vi "array -- find interval - real.vi"(8 "number":dbl, 11 "array":dbl[](array[numeric])=[10.0, 20.0, 56.0, 92.0, 120.0, 183.0, 194.0, 310.0]) -> (0 "omega plus (kHz)":dbl, 1 "omega zero (kHz)":dbl, 2 "omega minus (kHz)":dbl, 3 "out of range?":bool, 4 "closest element index":i32, 5 "exact match ?":bool)   [LabVIEW 2015]
uses:
  comparison control.ctl
  Q - not nan -- real.vi
panel:
  out "selector":T1
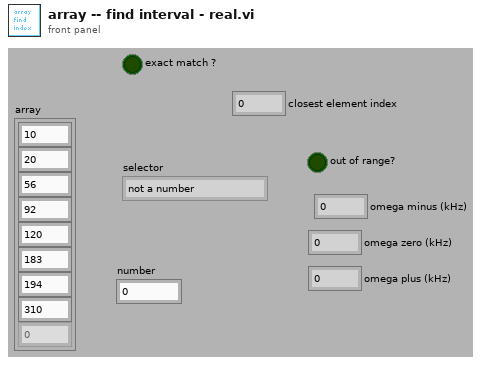
[diagram p1: front panel]
types:
  T1 = typedef "comparison control.ctl" = enum16{"not a number", "above", "in range", "below"}
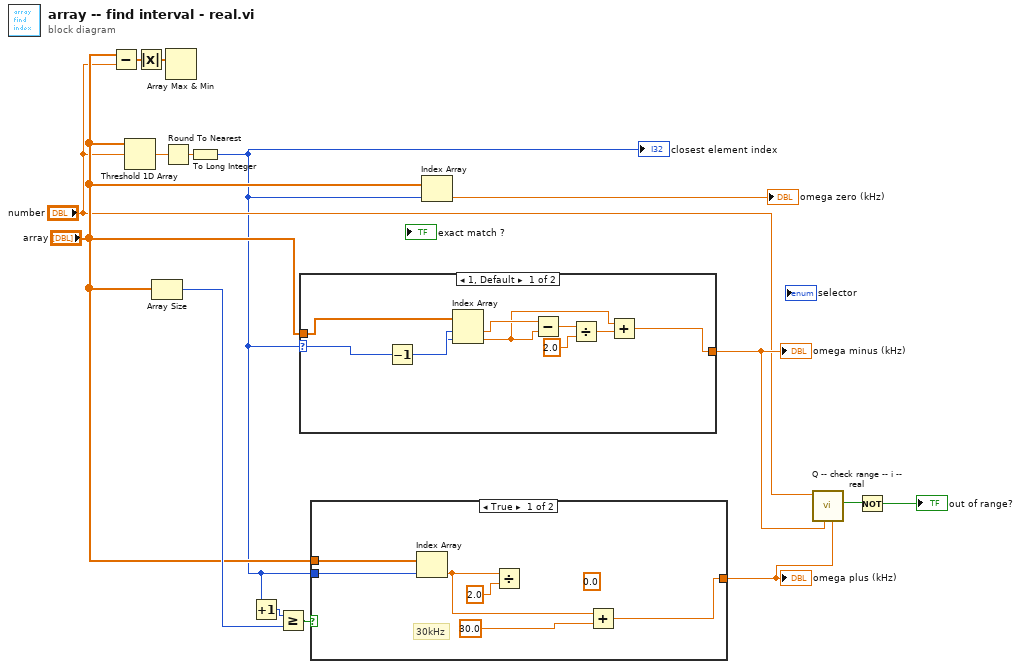
[diagram p0: block diagram]
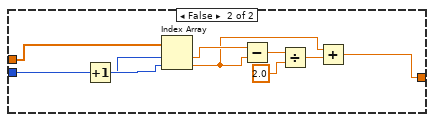
[diagram p2: hidden frame]
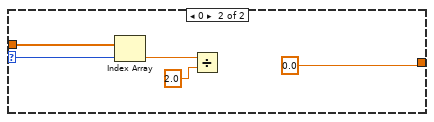
[diagram p3: hidden frame]
diagram:
  n1 = Subtract(x="array", y="number") -> (x-y=w7:dbl[])
  n2 = Threshold 1D Array(2:"number", 3:"array") -> (0:w3:dbl)  [unwired: 1 in]
  n3 = Absolute Value(x=w7) -> (abs(x)=w6:dbl[])
  n4 = Array Size(array="array") -> (size(s)=w13:i32)
  n5 = Round To Nearest(number=w3) -> (nearest integer value=w2:dbl)
  n6 = Array Max & Min(array=w6) -> ()  [unwired: 4 out]
  n7 = To Long Integer(number=w2) -> (32bit integer=w1:i32)
  "closest element index" <- w1
  n8 = Increment(x=w1) -> (x+1=w14:i32)
  n9 = Greater Or Equal?(x=w14, y=w13) -> (x >= y?=w12:bool)
  n10 = case shown="1, Default" w1 {
    selector: w1 -> [w20 w26]
    tunnel: "array" -> [w21 w27]
    tunnel: [w16 0.0] -> w11
    frame 1, Default {
      n11 = Decrement(x=w20) -> (x-1=w19:i32)
      n12 = Index Array(array=w21, index #1=w20, index #2=w19) -> (element #1=w18:dbl, element #2=w17:dbl)
      n13 = Subtract(x=w18, y=w17) -> (x-y=w24:dbl)
      n14 = Divide(x=w24, y=2.0) -> (x/y=w22:dbl)
      n15 = Add(x=w17, y=w22) -> (x+y=w16:dbl)
    }
    frame 0 {
      n16 = Index Array(array=w27, index=w26) -> (element=w28:dbl)
      n17 = Divide(x=w28, y=2.0) -> ()  [unwired: 1 out]
    }
  }
  "omega minus (kHz)" <- w11
  n18 = case shown="True" w12 {
    tunnel: "array" -> [w34 w41]
    tunnel: [w30 w38] -> w10
    tunnel: w1 -> [w32 w37]
    frame True {
      (unwired) 0.0
      # "30kHz"
      n19 = Index Array(array=w34, index=w32) -> (element=w31:dbl)
      n20 = Divide(x=w31, y=2.0) -> ()  [unwired: 1 out]
      n21 = Add(x=w31, y=30.0) -> (x+y=w30:dbl)
    }
    frame False {
      n22 = Increment(x=w37) -> (x+1=w36:i32)
      n23 = Index Array(array=w41, index #1=w36, index #2=w37) -> (element #1=w40:dbl, element #2=w39:dbl)
      n24 = Subtract(x=w40, y=w39) -> (x-y=w44:dbl)
      n25 = Divide(x=w44, y=2.0) -> (x/y=w42:dbl)
      n26 = Add(x=w39, y=w42) -> (x+y=w38:dbl)
    }
  }
  "omega plus (kHz)" <- w10
  n27 = Index Array(array="array", index=w1) -> (element=→"omega zero (kHz)":dbl)
  n28 = call "Q -- check range -- i -- real.vi"("upper"=w10, "lower"=w11, "number"="number") -> ("in range?"=w9:bool)  [unwired: 6 in, 2 out]
  n29 = Not(x=w9) -> (.not. x?=→"out of range?":bool)
